vi "PCert-Glue-Tree-ItemTypeToGlyph.vi"(0 "Item Type":string) -> (1 "All Icons":T1[](array[typedef]), 2 "Display Name":string, 3 "Glyph Index":i32)   [LabVIEW 2013]
uses:
  <vilib>/picture/picture.llb/imagedata.ctl
panel:
  # "Inputs"
  # "Outputs"
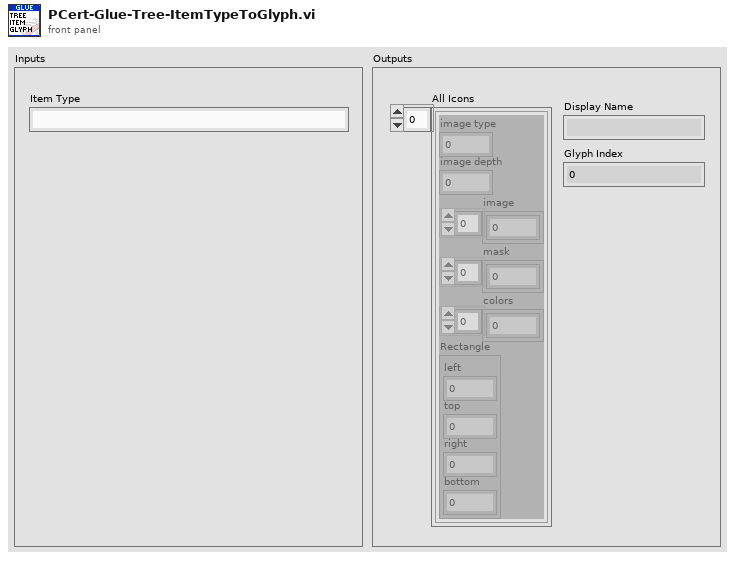
[diagram p1: front panel]
types:
  T1 = typedef "imagedata.ctl" = cluster{"image type":i32, "image depth":i32, "image":u8[], "mask":u8[], "colors":u32[], "Rectangle":cluster{"left":i16, "top":i16, "right":i16, "bottom":i16}}
  T2 = cluster{"UID":string, "Display Name":string, "Icon":T1, "Preview":picture}[]
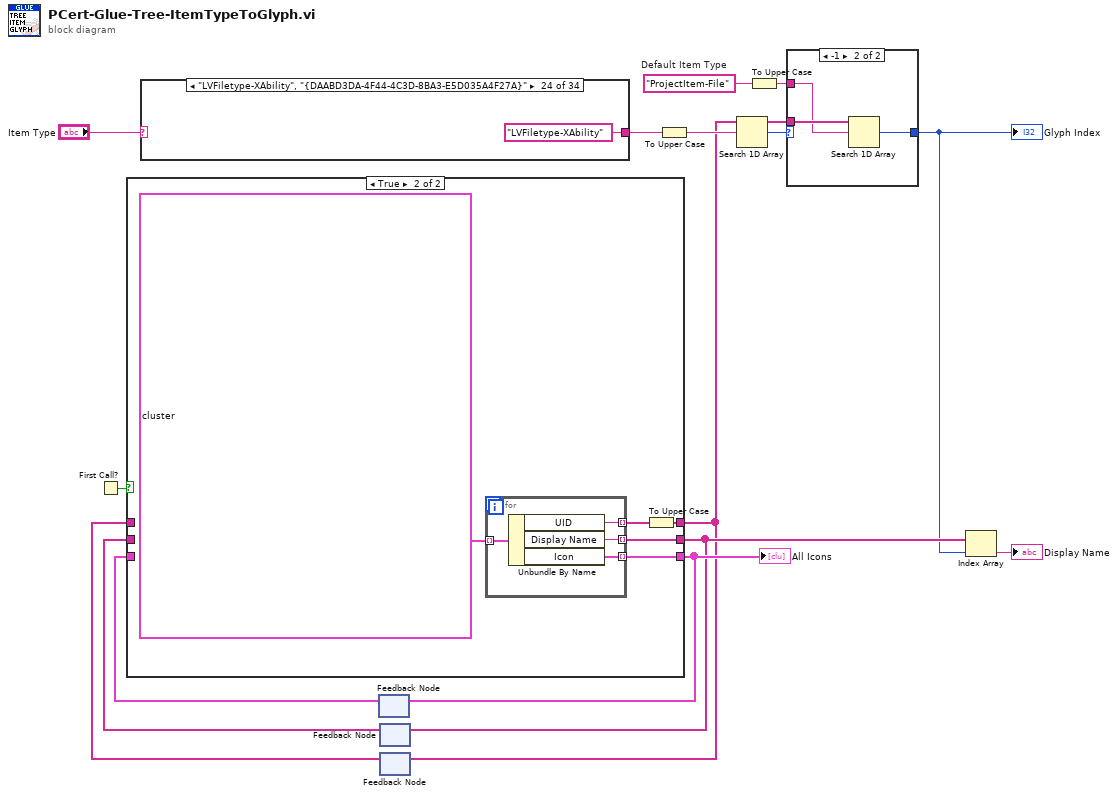
[diagram p0: block diagram]
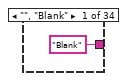
[diagram p4: hidden frame]
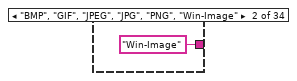
[diagram p5: hidden frame]
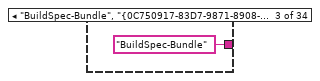
[diagram p6: hidden frame]
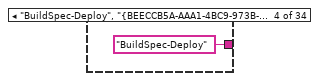
[diagram p7: hidden frame]
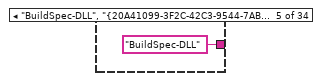
[diagram p8: hidden frame]
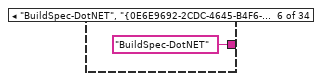
[diagram p9: hidden frame]
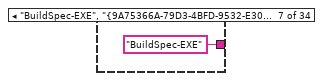
[diagram p10: hidden frame]
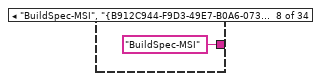
[diagram p11: hidden frame]
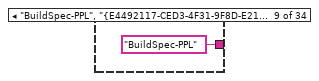
[diagram p12: hidden frame]
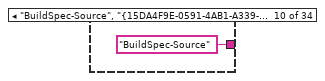
[diagram p13: hidden frame]
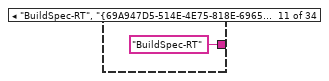
[diagram p14: hidden frame]
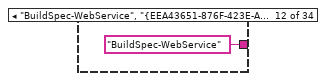
[diagram p15: hidden frame]
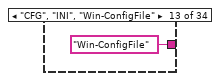
[diagram p16: hidden frame]
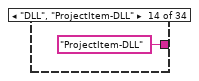
[diagram p17: hidden frame]
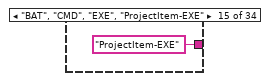
[diagram p18: hidden frame]
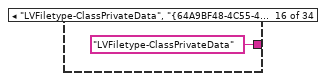
[diagram p19: hidden frame]
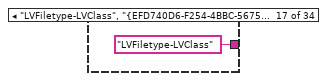
[diagram p20: hidden frame]
diagram:
  w2 = "ProjectItem-File"  # Default Item Type
  n1 = First Call?() -> (First Call?: T/F=w15:bool)
  n2 = case shown="\"LVFiletype-XAbility\", \"{DAABD3DA-4F44-4C3D-8BA3-E5D035A4F27A}\"" "Item Type" {
    selector: "Item Type" -> [_ _ _ _ _ _ _ _ _ _ _ _ _ _ _ _ _ _ _ _ _ _ _ _ _ _ _ _ _ _ _ _ _ w49]
    tunnel: ["Blank" ("Display Name") "Win-Image" ("Display Name") "BuildSpec-Bundle" ("Display Name") "BuildSpec-Deploy" ("Display Name") "BuildSpec-DLL" ("Display Name") "BuildSpec-DotNET" ("Display Name") "BuildSpec-EXE" ("Display Name") "BuildSpec-MSI" ("Display Name") "BuildSpec-PPL" ("Display Name") "BuildSpec-Source" ("Display Name") "BuildSpec-RT" ("Display Name") "BuildSpec-WebService" ("Display Name") "Win-ConfigFile" ("Display Name") "ProjectItem-DLL" ("Display Name") "ProjectItem-EXE" ("Display Name") "LVFiletype-ClassPrivateData" ("Display Name") "LVFiletype-LVClass" ("Display Name") "LVFiletype-LVLIB" ("Display Name") "LVFiletype-LVLIBP" ("Display Name") "LVFiletype-LVProj" ("Display Name") "LVFiletype-NSVariable" ("Display Name") "LVFiletype-PropertyFolder" ("Display Name") "LVFiletype-VI" ("Display Name") "LVFiletype-XAbility" ("Display Name") "LVFiletype-XControl" ("Display Name") "LVFiletype-XProperty" ("Display Name") "ProjectItem-Dependency" ("Display Name") "ProjectItem-File" ("Display Name") "ProjectItem-Folder" ("Display Name") "ProjectItem-MyComputer" ("Display Name") "ProjectItem-TXT" ("Display Name") "Win-Zip" ("Display Name") "LVFiletype-XProperty" ("Display Name") w49] -> w8
    frame "", "Blank" {
    }
    frame "BMP", "GIF", "JPEG", "JPG", "PNG", "Win-Image" {
    }
    frame "BuildSpec-Bundle", "{0C750917-83D7-9871-8908-BB4ED6A8099B}" {
    }
    frame "BuildSpec-Deploy", "{BEECCB5A-AAA1-4BC9-973B-EDB26338DA05}" {
    }
    frame "BuildSpec-DLL", "{20A41099-3F2C-42C3-9544-7ABCC1E6CB0D}" {
    }
    frame "BuildSpec-DotNET", "{0E6E9692-2CDC-4645-B4F6-93F9260BF6FA}" {
    }
    frame "BuildSpec-EXE", "{9A75366A-79D3-4BFD-9532-E3070185C1E8}" {
    }
    frame "BuildSpec-MSI", "{B912C944-F9D3-49E7-B0A6-073ED50A150B}" {
    }
    frame "BuildSpec-PPL", "{E4492117-CED3-4F31-9F8D-E2118AE04F12}" {
    }
    frame "BuildSpec-Source", "{15DA4F9E-0591-4AB1-A339-C3B4D54902D8}" {
    }
    frame "BuildSpec-RT", "{69A947D5-514E-4E75-818E-69657C0547D8}" {
    }
    frame "BuildSpec-WebService", "{EEA43651-876F-423E-A4A2-E7685CF2A672}" {
    }
    frame "CFG", "INI", "Win-ConfigFile" {
    }
    frame "DLL", "ProjectItem-DLL" {
    }
    frame "BAT", "CMD", "EXE", "ProjectItem-EXE" {
    }
    frame "LVFiletype-ClassPrivateData", "{64A9BF48-4C55-45DB-8F18-9C796DA0C113}" {
    }
    frame "LVFiletype-LVClass", "{EFD740D6-F254-4BBC-5675-8858F35B820E}" {
    }
    frame "LVFiletype-LVLIB", "{ABC740D6-F254-4BBC-5675-8858F35B820E}" {
    }
    frame "LVFiletype-LVLIBP", "{CF31838A-5E97-4315-AE50-9EBA613BCBBB}" {
    }
    frame "LVFiletype-LVProj", "{D60740D6-F254-4BBC-9975-8858F35B810E}" {
    }
    frame "LVFiletype-NSVariable", "{9BA597C5-4996-4622-B9BB-444431834D0D}" {
    }
    frame "LVFiletype-PropertyFolder", "{93C4A07A-46E9-442F-AF0F-D6C6039546D1}" {
    }
    frame "LVFiletype-VI", "{D60740D6-F254-4BBC-5675-8858F35B810E}" {
    }
    frame "LVFiletype-XAbility", "{DAABD3DA-4F44-4C3D-8BA3-E5D035A4F27A}" {
    }
    frame "LVFiletype-XControl", "{2E4BD3AC-4E04-45C9-B6C5-AD138962C435}" {
    }
    frame "LVFiletype-XProperty", "{81C68620-8BE3-4643-B04A-4E83AA6363D2}" {
    }
    frame "ProjectItem-Dependency", "{0D75D917-83D7-9871-AA09-A0FFD6A8099B}" {
    }
    frame "ProjectItem-File", "{D60740D6-F255-4BBC-5675-8858F35B820E}" {
    }
    frame "ProjectItem-Folder", "{D60740D6-F254-4BBC-5675-8858F35B820E}" {
    }
    frame "ProjectItem-MyComputer", "{CEFE1B10-1732-4678-A70A-299293455410}" {
    }
    frame "ProjectItem-TXT", "RTF", "TXT" {
    }
    frame "Win-Zip", "{51F0E16F-7FA4-4E9F-AE30-C81D9D0444B0}" {
    }
    frame "{DAABD3DB-4F44-4C3D-8BA3-E5D035A4F27A}" {
    }
    frame Default {
    }
  }
  n3 = feedback #1() -> (w13:T1[])  [unwired: 1 in]
  n4 = feedback #2() -> (w12:string[])  [unwired: 1 in]
  n5 = feedback #3() -> (w11:string[])  [unwired: 1 in]
  n6 = case shown="True" w15 {
    tunnel: [w50 w54] -> w4
    tunnel: [w51 w56] -> w7
    tunnel: [w52 w55] -> w14
    tunnel: w13 -> [w52 _]
    tunnel: w12 -> [w51 _]
    tunnel: w11 -> [w50 _]
    frame False {
    }
    frame True {
      n7 = for {
        tunnel: T2 data[167230B] ("Array") -> [w61] mode=indexing
        tunnel: [w60] -> w57 mode=indexing
        tunnel: [w59] -> w56 mode=indexing
        tunnel: [w58] -> w55 mode=indexing
        n8 = Unbundle By Name(w61) -> ("UID"=w60:string, "Display Name"=w59:string, "Icon"=w58:T1)
      }
      n9 = To Upper Case(1:w57) -> (0:w54:string[])
    }
  }
  "All Icons" <- w14
  n10 = feedback-in #1(w14) -> ()
  n11 = feedback-in #2(w7) -> ()
  n12 = feedback-in #3(w4) -> ()
  n13 = To Upper Case(1:w8) -> (0:w10:string)
  n14 = Search 1D Array(1D array=w4, element=w10) -> (index of element=w5:i32)  [unwired: 1 in]
  n15 = To Upper Case(1:w2) -> (0:w1:string)
  n16 = case shown="-1" w5 {
    selector: w5 -> [w62 _]
    tunnel: w4 -> [_ w65]
    tunnel: [w62 w64] -> w3
    tunnel: w1 -> [_ w63]
    frame Default {
    }
    frame -1 {
      n17 = Search 1D Array(1D array=w65, element=w63) -> (index of element=w64:i32)  [unwired: 1 in]
    }
  }
  "Glyph Index" <- w3
  n18 = Index Array(array=w7, index=w3) -> (element=→"Display Name":string)
